vi "oa_Simple Sample Rate Conversion (Continuous) (N Channels).vi"(7 "reset? (T)":bool=TRUE, 8 "even angle position info":T1, 9 "interpolation mode":u16(ring)=1 items=["coerce", "linear", "spline", "FIR filter"], 10 "dr":dbl=1.0 format="%.2p", 11 "even angle signals":cluster{"r0":dbl, "dr":dbl, "Y":dbl[]}[](array[cluster]) {"r0" format="%.2p"; "dr" format="%.2p"; "Y" format="%.2f"}) -> (0 "error out":errorcluster, 2 "out even angle position info":T1, 3 "even angle signals out":cluster{"r0":dbl, "dr":dbl, "Y":dbl[]}[](array[cluster]) {"r0" format="%.2p"; "dr" format="%.2p"; "Y" format="%.2f"})   [LabVIEW 2017, in "SoundVib_OAUtility.lvlib"]
uses:
  <vilib>/addons/Sound and Vibration/Order Analysis/Utility/SoundVib_OAUtility.lvlib
  <vilib>/addons/Sound and Vibration/Order Analysis/Misc/OAT Position Info.ctl
  <vilib>/measure/maresamp.llb/Resample Waveform (continuous, t0 DBL).vi
  <vilib>/measure/maresamp.llb/Resample N Waveforms (continuous, t0 DBL).vi
  <vilib>/measure/NI_MAPro.lvlib
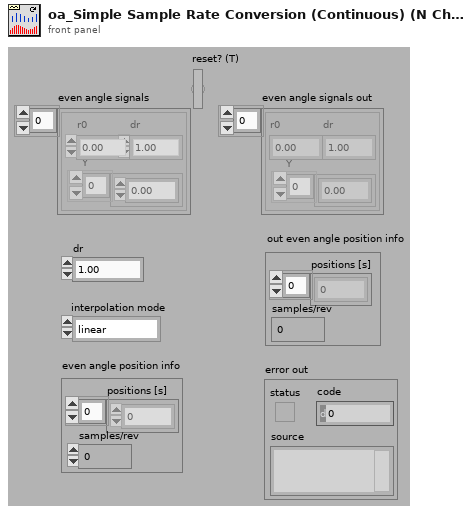
[diagram p1: front panel]
types:
  T1 = typedef "OAT Position Info.ctl" = cluster{"positions [s]":dbl[], "samples/rev":dbl}
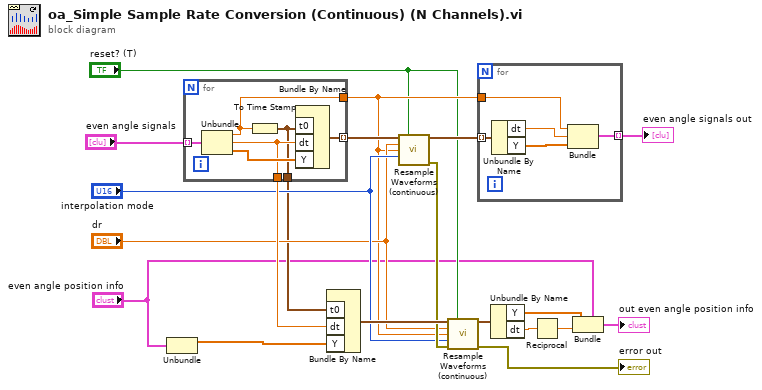
[diagram p0: block diagram]
diagram:
  n1 = Unbundle("even angle position info") -> ("positions [s]"=w3:dbl[])  [unwired: 1 out]
  n2 = for {
    tunnel: [w26] -> w20 mode=indexing
    tunnel: [w24] -> w13
    tunnel: [w23] -> w10
    tunnel: [w22] -> w6
    tunnel: "even angle signals" -> [w21] mode=indexing
    n3 = Unbundle(w21) -> ("r0"=w23:dbl, "dr"=w24:dbl, "Y"=w25:dbl[])
    n4 = To Time Stamp(1:w23) -> (0:w22:timestamp)
    n5 = Bundle By Name("t0"=w22, "dt"=w24, "Y"=w25) -> (w26:waveform(dbl))  [unwired: 1 in]
  }
  n6 = Bundle By Name("t0"=w6, "dt"=w13, "Y"=w3) -> (w18:waveform(dbl))  [unwired: 1 in]
  n7 = call-poly <vilib>:"Resample Waveforms (continuous).vi"("waveforms in"=w20, "reset"="reset? (T)", "dt"="dr", "t0"=w10, "interpolation mode"="interpolation mode") -> ("resampled waveforms out"=w19:waveform(dbl)[], "error out"=w17:errorcluster)  [unwired: 6 in, 3 out]
  n8 = call-poly <vilib>:"Resample Waveforms (continuous).vi"("waveform in"=w18, "reset"="reset? (T)", "dt"="dr", "t0"=w10, "interpolation mode"="interpolation mode", "error in (no error)"=w17) -> ("resampled waveform out"=w16:waveform(dbl), "error out"=→"error out":errorcluster)  [unwired: 5 in, 3 out]
  n9 = for {
    tunnel: w19 -> [w31] mode=indexing
    tunnel: w10 -> [w28]
    tunnel: [w27] -> w1 mode=indexing
    n10 = Unbundle By Name(w31) -> ("dt"=w30:dbl, "Y"=w29:dbl[])
    n11 = Bundle("r0"=w28, "dt"=w30, "Y"=w29) -> (w27:cluster{"r0":dbl, "dt":dbl, "Y":dbl[]})  [unwired: 1 in]
  }
  "even angle signals out" <- w1
  n12 = Unbundle By Name(w16) -> ("Y"=w8:dbl[], "dt"=w15:dbl)
  n13 = Reciprocal(x=w15) -> (1/x=w14:dbl)
  n14 = Bundle(cluster="even angle position info", "positions [s]"=w8, "samples/rev"=w14) -> (→"out even angle position info":T1)
